vi "F Dwf Get Last Error Msg.vi"(8 "error in (no error)":errorcluster, 11 "szError":string) -> (0 "error out":errorcluster, 2 "function return":i32, 3 "szError out":string)   [LabVIEW 2019, in "Olasdwf.lvlib"]
doc: "DWFAPI int FDwfGetLastErrorMsg(char szError[512]);"
uses:
  Olasdwf.lvlib
  Windows/System32/dwf.dll
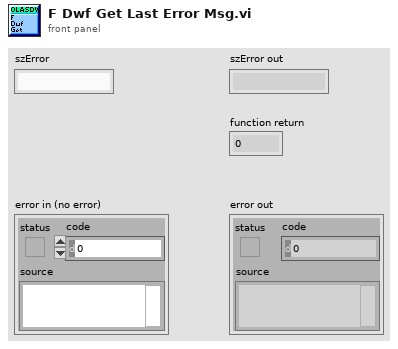
[diagram p1: front panel]
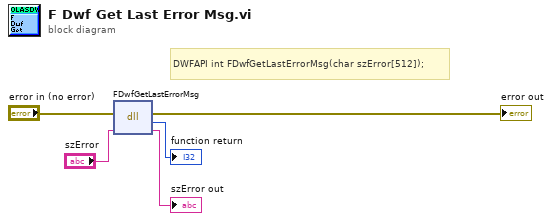
[diagram p0: block diagram]
diagram:
  # "DWFAPI int FDwfGetLastErrorMsg(char szError[512]);"
  n1 = dll-call lib="C:/Windows/System32/dwf.*" fn="FDwfGetLastErrorMsg"(error in="error in (no error)", "szError"="szError") -> (error out=→"error out":errorcluster, →"function return":i32, "szError"=→"szError out":string)  [unwired: 2 in, 1 out]
